vi "Auto Turn.vi"(9 "Turn Amount":dbl=8.0 format="%#_13g", 10 "+/-?":dbl, 11 "Run?":bool) -> (3 "Done":bool)   [LabVIEW 2013]
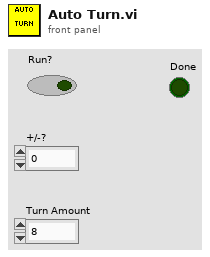
[diagram p1: front panel]
types:
  T1 = typedef "WPI_I2CDevRef.ctl" = cluster{"DevStatus":errorcluster, "Digital Module":T2, "Device Address":u8}
  T2 = typedef "FPGA_TypedefDigitalModule.ctl" = enum16{"Digital Module 1", "Digital Module 2"}
  T3 = typedef "WPI_MotorControlDeviceRef.ctl" = cluster{"DeviceStatus":errorcluster, "Type":enum16{"PWM", "CAN"}, "PWM":cluster{"Digital Module":T2, "PWM Channel":T4, "DeadBand":T5}, "CAN":cluster{"Device Number":u8, "Control Mode":T6, "Semaphore":T7, "Max Vout":dbl}, "Invert":bool, "TransformRef":T8, "InvTransformRef":T8}
  T4 = typedef "FPGA_DIOPWMChannel.ctl" = enum8{"PWM 1", "PWM 2", "PWM 3", "PWM 4", "PWM 5", "PWM 6", "PWM 7", "PWM 8", "PWM 9", "PWM 10", "Invalid"}
  T5 = typedef "WPI_PWMDeadband.ctl" = cluster{"Name":string, "maxPositivePwm":i32, "minPositivePwm":i32, "centerPwm":i32, "maxNegativePwm":i32, "minNegativePwm":i32, "angularRange":u16}
  T6 = typedef "WPI_CANJaguar_ControlMode.ctl" = enum8{"Percent VBus", "Current", "Speed", "Position", "Voltage"}
  T7 = typedef "Semaphore RefNum" = refnum<k1>
  T8 = typedef "WPI_PWMTransform_ConPane.ctl" = refnum<vi>
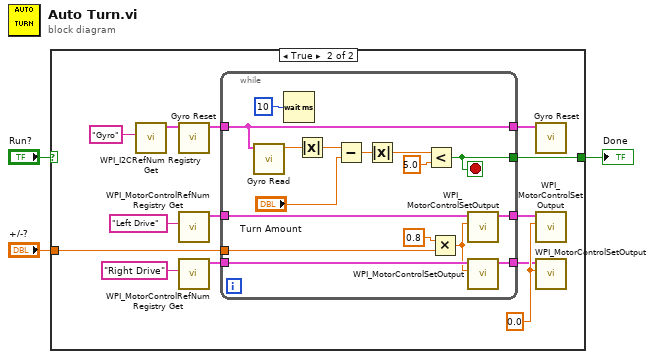
[diagram p0: block diagram]
diagram:
  n1 = case shown="True" "Run?" {
    selector: "Run?" -> [w4 _]
    tunnel: [w4 w7] -> w2
    tunnel: "+/-?" -> [_ w6]
    frame False {
    }
    frame True {
      w17 = 0.0 ("Output")
      n2 = call <vilib>:"WPI_I2CRefNum Registry Get.vi"("refnum name"="Gyro") -> ("I2CDevRef"=w13:T1)  [unwired: 9 in, 1 out]
      n3 = call "Gyro Reset.vi"("I2CDevRef"=w13) -> ("I2CDevRef Out"=w14:T1)  [unwired: 10 in]
      n4 = call <vilib>:"WPI_MotorControlRefNum Registry Get.vi"("refnum name"="Left Drive") -> ("MotorControlDevRef"=w9:T3)  [unwired: 9 in, 1 out]
      n5 = call <vilib>:"WPI_MotorControlRefNum Registry Get.vi"("refnum name"="Right Drive") -> ("MotorControlDevRef"=w8:T3)  [unwired: 9 in, 1 out]
      n6 = while {
        tunnel: w14 -> [w18]
        tunnel: w9 -> [w29]
        tunnel: w8 -> [w28]
        tunnel: w6 -> [w24]
        tunnel: [w21] -> w15
        tunnel: [w20] -> w16
        tunnel: [w19] -> w7
        tunnel: [w18] -> w5
        stop <- w19 stop-if-true
        n7 = call "Gyro Read.vi"("I2CDevRef In"=w18) -> ("Angle"=w32:dbl)  [unwired: 9 in, 1 out]
        n8 = Wait (ms)(milliseconds to wait=u32 10) -> ()  [unwired: 1 out]
        n9 = Absolute Value(x=w32) -> (abs(x)=w25:dbl)
        n10 = Subtract(x=w25, y="Turn Amount") -> (x-y=w30:dbl)
        n11 = Absolute Value(x=w30) -> (abs(x)=w27:dbl)
        n12 = Less?(x=w27, y=5.0) -> (x < y?=w19:bool)
        n13 = Multiply(x=0.8 ("Output"), y=w24) -> (x*y=w22:dbl)
        n14 = call <vilib>:"WPI_MotorControlSetOutput.vi"("Output"=w22, "MotorControlDevRef"=w29) -> ("MotorControlDevRef"=w20:T3)  [unwired: 7 in, 2 out]
        n15 = call <vilib>:"WPI_MotorControlSetOutput.vi"("Output"=w22, "MotorControlDevRef"=w28) -> ("MotorControlDevRef"=w21:T3)  [unwired: 7 in, 2 out]
      }
      n16 = call "Gyro Reset.vi"("I2CDevRef"=w5) -> ()  [unwired: 10 in, 1 out]
      n17 = call <vilib>:"WPI_MotorControlSetOutput.vi"("Output"=w17, "MotorControlDevRef"=w16) -> ()  [unwired: 7 in, 3 out]
      n18 = call <vilib>:"WPI_MotorControlSetOutput.vi"("Output"=w17, "MotorControlDevRef"=w15) -> ()  [unwired: 7 in, 3 out]
    }
  }
  "Done" <- w2
